vi "example async loop.vi"() -> ()   [LabVIEW 2016]
panel:
  out "data1 2":u32
  out "data1":u32
  out "packetType":T1(ring)
  out "System Index":u32
  in  "Channel":u32
  in  "Position Difference [nm]":i32=8000
  out "Error":errorcluster
  out "State":enum16{"POLL", "IDLE", "START", "RUN", "STOP"}(ring)
  in  "abort":bool
  out "Exit":bool
  out "connected":bool
  in  "connect":bool
  in  "findSystems":bool caption="Find Systems"
  in  "System locator":string(combo)
  in  "start":bool
  # "A linear positioner with integrated sensor \nshould be connected to channel 0."
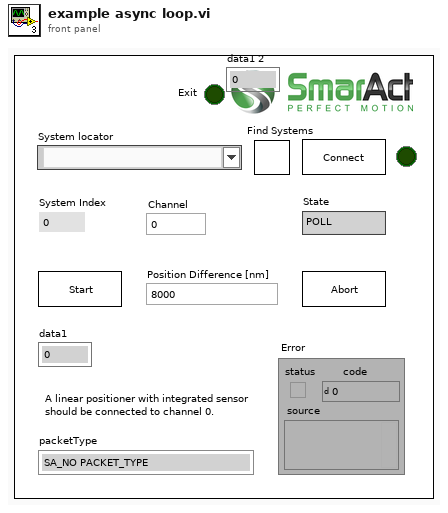
[diagram p1: front panel]
types:
  T1 = enum32{"SA_NO PACKET_TYPE", "SA_ERROR_ PACKET_TYPE", "SA_POSITION PACKET_TYPE", "SA_COMPLETED PACKET_TYPE", "SA_STATUS PACKET_TYPE", "SA_ANGLE_PACKET_TYPE", "SA_VOLTAGE_LEVEL_PACKET_TYPE", "SA_SENSOR_TYPE_PACKET_TYPE", "SA_SENSOR_ENABLED_PACKET_TYPE", "SA_END_EFFECTOR_TYPE_PACKET_TYPE", "SA_GRIPPER_OPENING_PACKET_TYPE", "SA_FORCE_PACKET_TYPE", "SA_MOVE_SPEED_PACKET_TYPE", "SA_PHYSICAL_POSITION_KNOWN_PACKET_TYPE", "SA_POSITION_LIMIT_PACKET_TYPE", "SA_ANGLE_LIMIT_PACKET_TYPE", "SA_SAFE_DIRECTION_PACKET_TYPE", "SA_SCALE_PACKET_TYPE", "SA_MOVE_ACCELERATION_PACKET_TYPE", "SA_CHANNEL_PROPERTY_PACKET_TYPE", "SA_CAPTURE_BUFFER_PACKET_TYPE", "SA_TRIGGERED_PACKET_TYPE"}
  T2 = enum32{"SA_NO_REPORT_ON_COMPLETE", "SA_REPORT_ON_COMPLETE"}
  T3 = enum32{"SA_SENSOR_DISABLED", "SA_SENSOR_ENABLED", "SA_SENSOR_POWERSAVE"}
  T4 = enum32{"SA_UNBUFFERED_OUTPUT", "SA_BUFFERED_OUTPUT"}
  T5 = typedef "mcsPacket.ctl" = cluster{"packetType":enum32{"SA_NO PACKET_TYPE", "SA_ERROR_ PACKET_TYPE", "SA_POSITION PACKET_TYPE", "SA_COMPLETED PACKET_TYPE", "SA_STATUS PACKET_TYPE", "SA_ANGLE_PACKET_TYPE", "SA_VOLTAGE_LEVEL_PACKET_TYPE", "SA_SENSOR_TYPE_PACKET_TYPE", "SA_SENSOR_ENABLED_PACKET_TYPE", "SA_END_EFFECTOR_TYPE_PACKET_TYPE", "SA_GRIPPER_OPENING_PACKET_TYPE", "SA_FORCE_PACKET_TYPE", "SA_MOVE_SPEED_PACKET_TYPE", "SA_PHYSICAL_POSITION_KNOWN_PACKET_TYPE", "SA_POSITION_LIMIT_PACKET_TYPE", "SA_ANGLE_LIMIT_PACKET_TYPE", "SA_SAFE_DIRECTION_PACKET_TYPE", "SA_SCALE_PACKET_TYPE", "SA_MOVE_ACCELERATION_PACKET_TYPE", "SA_CHANNEL_PROPERTY_PACKET_TYPE", "SA_CAPTURE_BUFFER_PACKET_TYPE", "SA_TRIGGERED_PACKET_TYPE"}, "channelIndex":u32, "data1":u32, "data2":i32, "data3":i32, "data4":u32}
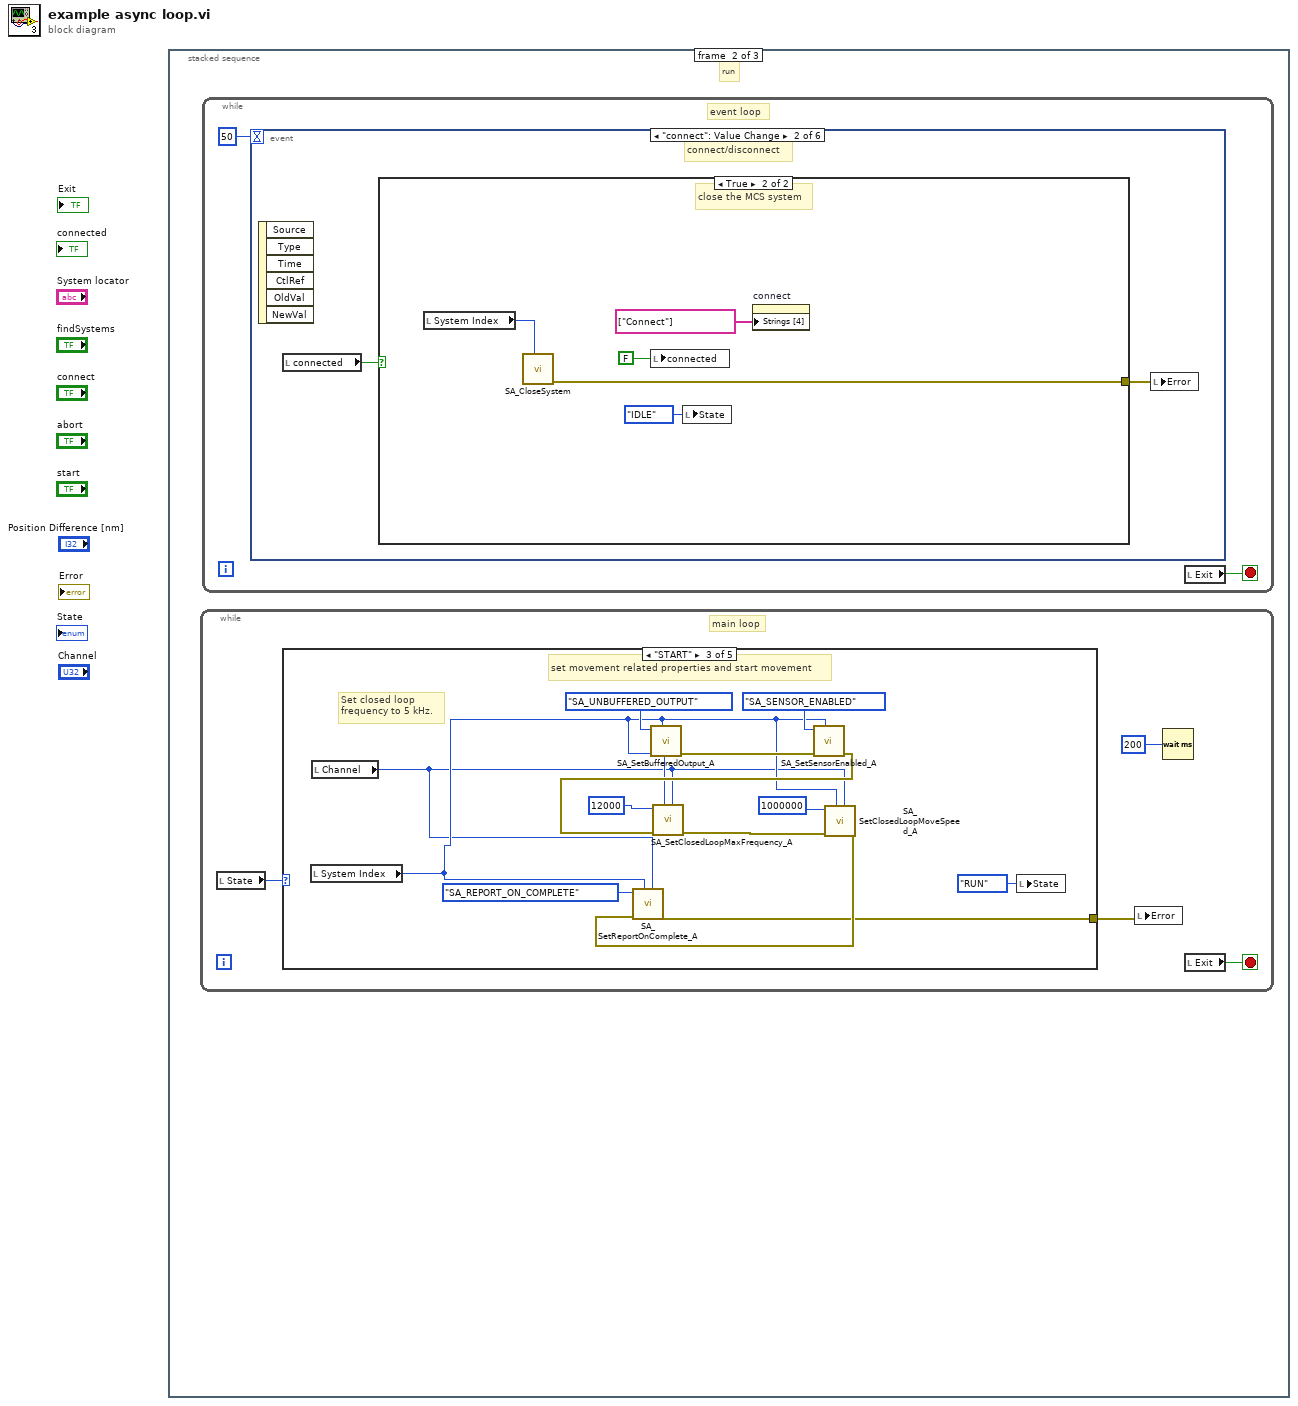
[diagram p0: block diagram]
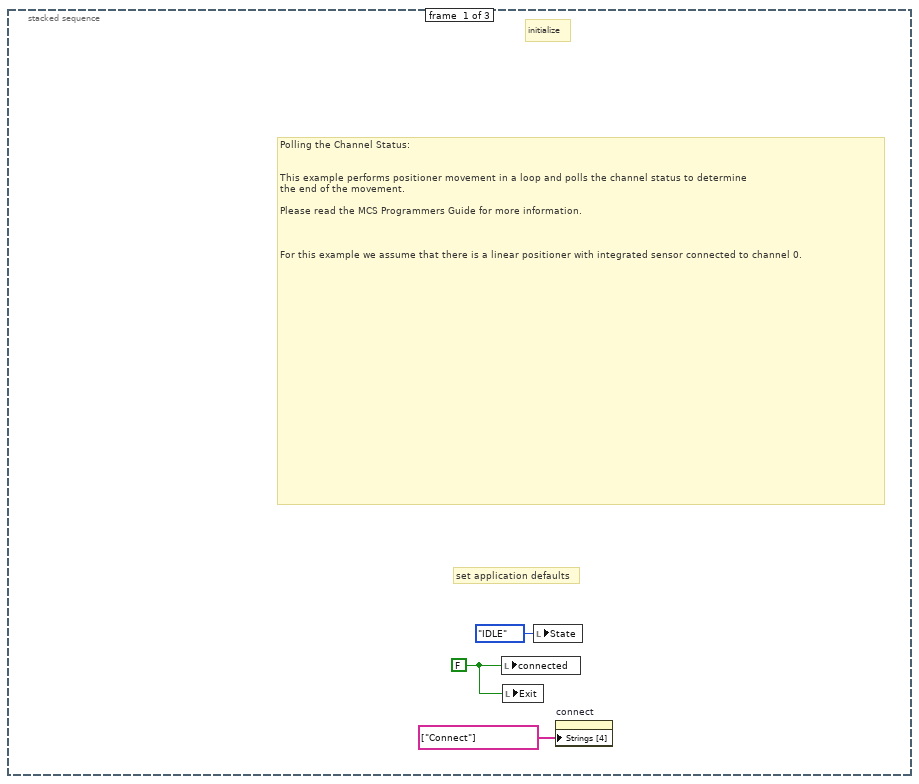
[diagram p2: hidden frame]
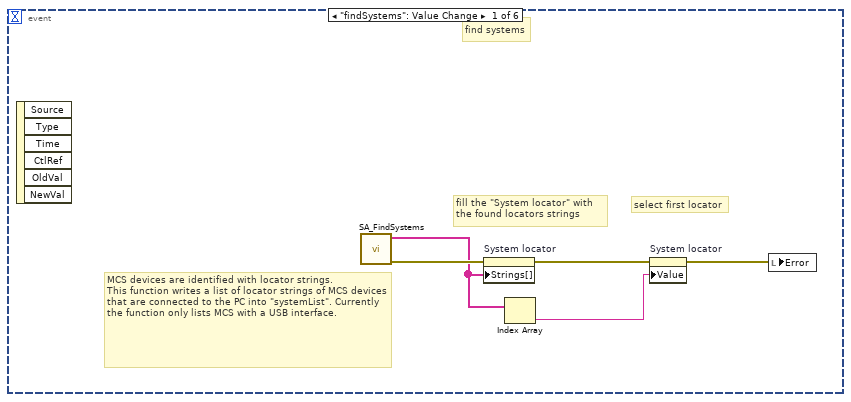
[diagram p3: hidden frame]
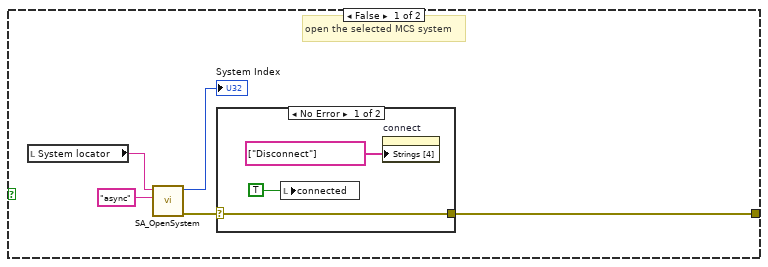
[diagram p4: hidden frame]
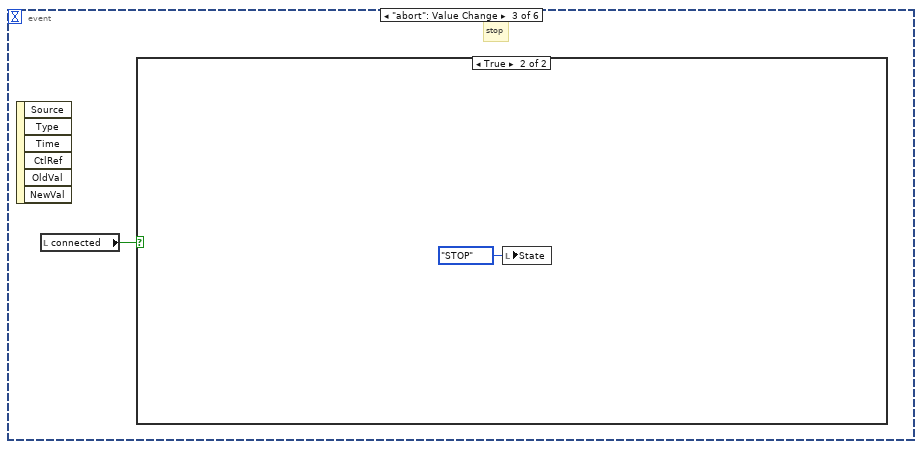
[diagram p6: hidden frame]
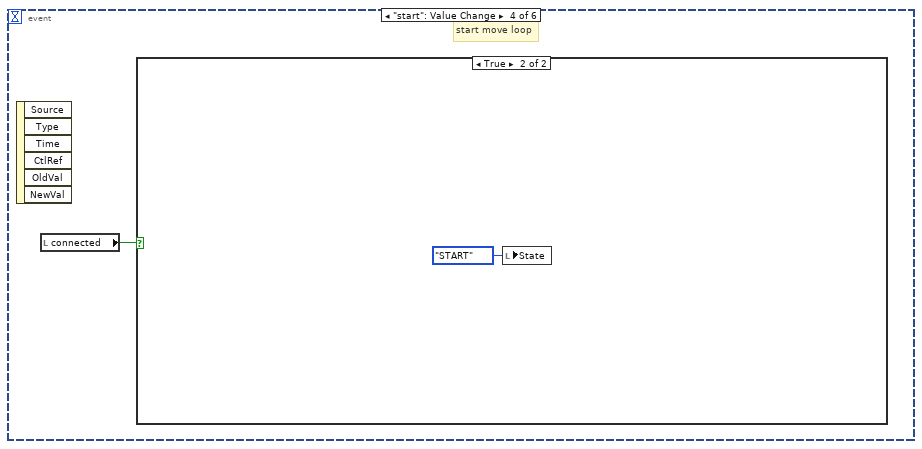
[diagram p8: hidden frame]
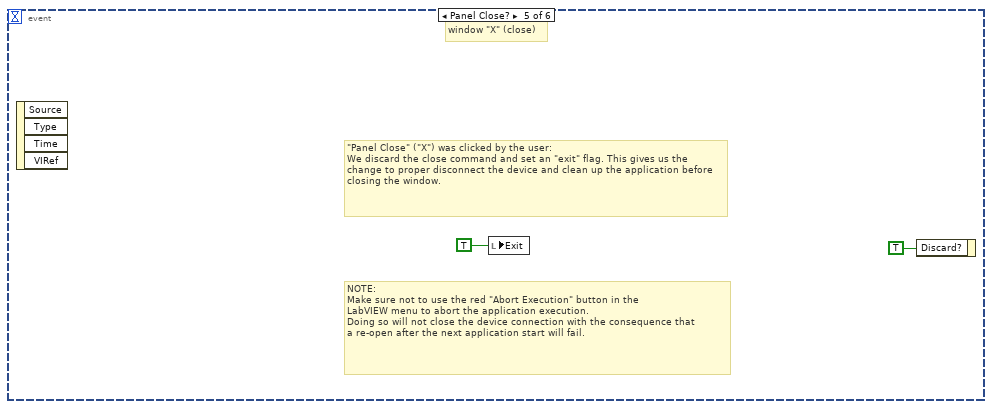
[diagram p10: hidden frame]
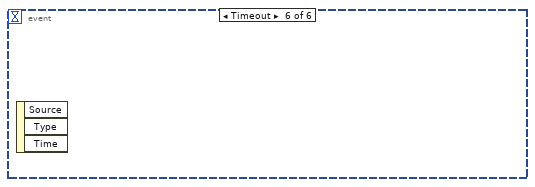
[diagram p11: hidden frame]
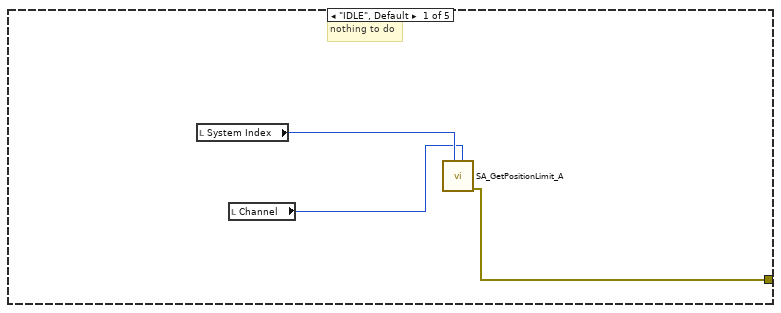
[diagram p12: hidden frame]
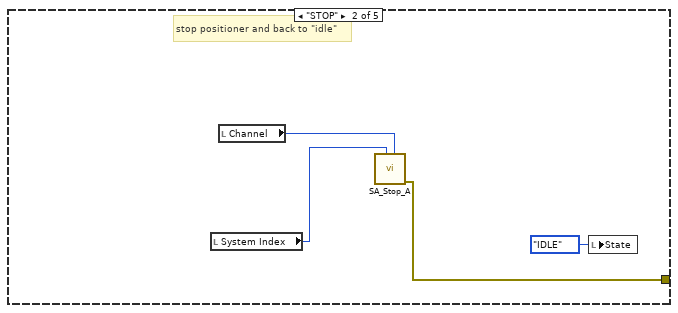
[diagram p13: hidden frame]
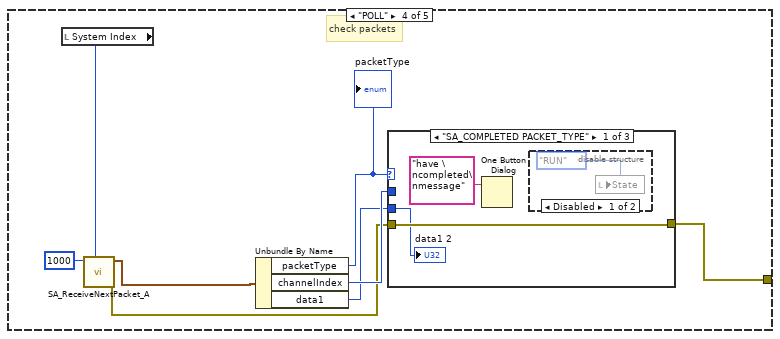
[diagram p14: hidden frame]
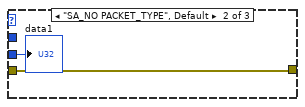
[diagram p16: hidden frame]
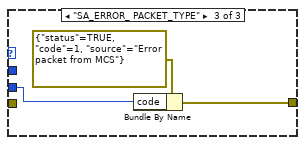
[diagram p17: hidden frame]
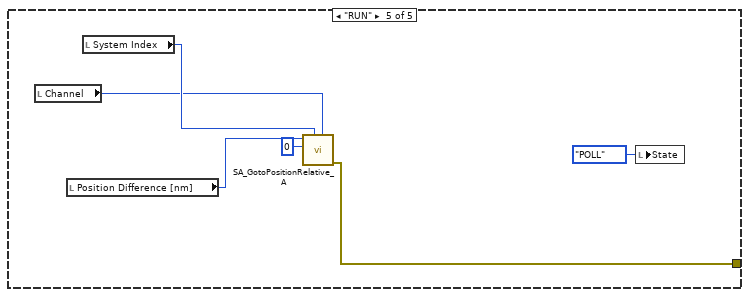
[diagram p18: hidden frame]
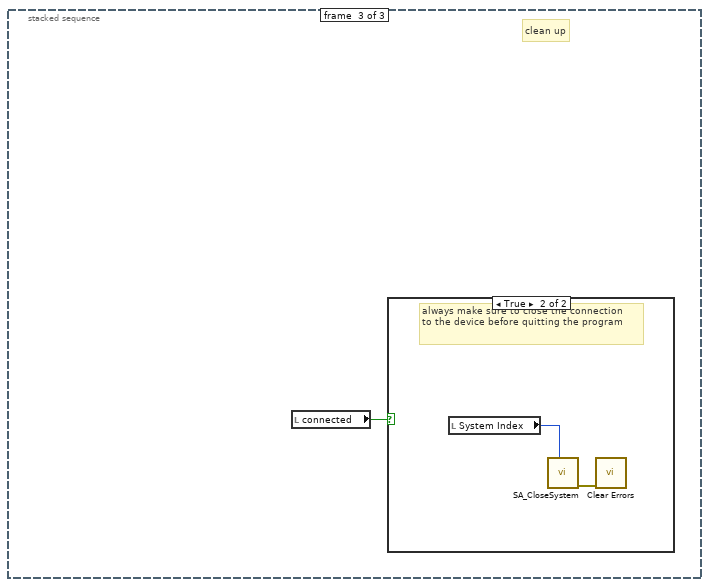
[diagram p19: hidden frame]
diagram:
  n1 = stacked-sequence {
    frame #0 {
      w3 = FALSE ("connected")
      # "Polling the Channel Status:\n\n\nThis example performs positioner movement in a loop and polls the channel status to determine\nthe end of the movement.\n\nPlease read the MCS Programmers Guide for more information.\n\n\n\nFor this example we assume that there is a linear positioner with integrated sensor connected to channel 0."
      # "set application defaults"
      # "initialize"
      n2 = local write "connected"(w3) -> ()
      n3 = local write "Exit"(w3) -> ()
      n4 = local write "State"(enum16{"POLL", "IDLE", "START", "RUN", "STOP"}."IDLE" ("State")) -> ()
      n5 = property on="connect" class="Bool"("Strings [4]"=string[] ["Connect"]) -> ()  [unwired: 2 in, 2 out]
    }
    frame #1 {
      # "run"
      n6 = while {
        stop <- w36 stop-if-true
        # "main loop"
        n7 = local read "State"() -> (w34:enum16{"POLL", "IDLE", "START", "RUN", "STOP"})
        n8 = case shown="\"START\"" w34 {
          tunnel: [w37 w42 w44 w58 w75] -> w33
          frame "IDLE", Default {
            # "nothing to do"
            n9 = local read "System Index"() -> (w39:u32)
            n10 = local read "Channel"() -> (w38:u32)
            n11 = call <vilib>:"SA_GetPositionLimit_A.vi"("channelIndex"=w38, "systemIndex"=w39) -> ("error out"=w37:errorcluster)  [unwired: 9 in]
          }
          frame "STOP" {
            # "stop positioner and back to \"idle\""
            n12 = local read "System Index"() -> (w41:u32)
            n13 = local read "Channel"() -> (w40:u32)
            n14 = call <vilib>:"SA_Stop_A.vi"("channelIndex"=w40, "systemIndex"=w41) -> ("error out"=w42:errorcluster)  [unwired: 9 in]
            n15 = local write "State"(enum16{"POLL", "IDLE", "START", "RUN", "STOP"}."IDLE" ("State")) -> ()
          }
          frame "START" {
            # "Set closed loop frequency to 5 kHz."
            # "set movement related properties and start movement"
            n16 = local read "System Index"() -> (w47:u32)
            n17 = local read "Channel"() -> (w46:u32)
            n18 = call <vilib>:"SA_SetBufferedOutput_A.vi"("systemIndex"=w47, "mode"=T4."SA_UNBUFFERED_OUTPUT") -> ("error out"=w54:errorcluster)  [unwired: 9 in]
            n19 = call <vilib>:"SA_SetSensorEnabled_A.vi"("systemIndex"=w47, "error in (no error)"=w54, "enabled"=T3."SA_SENSOR_ENABLED") -> ("error out"=w50:errorcluster)  [unwired: 8 in]
            n20 = call <vilib>:"SA_SetClosedLoopMaxFrequency_A.vi"("channelIndex"=w46, "systemIndex"=w47, "error in (no error)"=w50, "frequency"=u32 12000) -> ("error out"=w52:errorcluster)  [unwired: 7 in]
            n21 = call <vilib>:"SA_SetClosedLoopMoveSpeed_A.vi"("channelIndex"=w46, "systemIndex"=w47, "error in (no error)"=w52, "speed"=u32 1000000) -> ("error out"=w45:errorcluster)  [unwired: 7 in]
            n22 = call <vilib>:"SA_SetReportOnComplete_A.vi"("channelIndex"=w46, "systemIndex"=w47, "error in (no error)"=w45, "report"=T2."SA_REPORT_ON_COMPLETE") -> ("error out"=w44:errorcluster)  [unwired: 7 in]
            n23 = local write "State"(enum16{"POLL", "IDLE", "START", "RUN", "STOP"}."RUN" ("State")) -> ()
          }
          frame "POLL" {
            # "check packets"
            n24 = local read "System Index"() -> (w63:u32)
            n25 = call <vilib>:"SA_ReceiveNextPacket_A.vi"("systemIndex"=w63, "timeout"=u32 1000) -> ("error out"=w57:errorcluster, "packet"=w62:T5)  [unwired: 8 in]
            n26 = Unbundle By Name(w62) -> ("packetType"=w61:T1, "channelIndex"=w60:u32, "data1"=w59:u32)
            "packetType" <- w61
            n27 = case shown="\"SA_COMPLETED PACKET_TYPE\"" w61 {
              tunnel: [w67 w70 w72] -> w58
              tunnel: w59 -> [w65 w69 w71]
              tunnel: w60 -> [_ _ _]
              tunnel: w57 -> [w67 w70 _]
              frame "SA_COMPLETED PACKET_TYPE" {
                n28 = One Button Dialog(message="have \ncompleted\nmessage") -> ()  [unwired: 1 in, 1 out]
                n29 = disable-structure shown="Disabled" {
                  frame Disabled {
                    n30 = local write "State"(enum16{"POLL", "IDLE", "START", "RUN", "STOP"}."RUN" ("State")) -> ()
                  }
                  frame Enabled {
                  }
                }
                "data1 2" <- w65
              }
              frame "SA_NO PACKET_TYPE", Default {
                "data1" <- w69
              }
              frame "SA_ERROR_ PACKET_TYPE" {
                n31 = Bundle By Name(cluster=errorcluster {"status"=TRUE, "code"=1, "source"="Error packet from MCS"} ("error out"), "code"=w71) -> (w72:errorcluster)
              }
            }
          }
          frame "RUN" {
            n32 = local read "Channel"() -> (w77:u32)
            n33 = local read "Position Difference [nm]"() -> (w76:i32)
            n34 = local read "System Index"() -> (w78:u32)
            n35 = call <vilib>:"SA_GotoPositionRelative_A.vi"("channelIndex"=w77, "systemIndex"=w78, "holdTime"=u32 0, "diff"=w76) -> ("error out"=w75:errorcluster)  [unwired: 7 in]
            n36 = local write "State"(enum16{"POLL", "IDLE", "START", "RUN", "STOP"}."POLL" ("State")) -> ()
          }
        }
        n37 = local write "Error"(w33) -> ()
        n38 = Wait (ms)(milliseconds to wait=u32 200) -> ()  [unwired: 1 out]
        n39 = local read "Exit"() -> (w36:bool)
      }
      n40 = while {
        stop <- w4 stop-if-true
        # "event loop"
        n41 = event shown="[1] \"connect\": Value Change" {
          selector: _ -> [_ _ _ _ _ _]
          dyn-events: _ -> [_ _ _ _ _ _]
          timeout: 50 -> [_ _ _ _ _ _]
          event "findSystems": Value Change {
            # "select first locator"
            # "fill the \"System locator\" with\nthe found locators strings"
            # "MCS devices are identified with locator strings.\nThis function writes a list of locator strings of MCS devices that are connected to the PC into \"systemList\". Currently the function only lists MCS with a USB interface."
            # "find systems"
            n42 = event-data() -> ()  [unwired: 1 in, 6 out]
            n43 = call <vilib>:"SA_FindSystems.vi"() -> ("error out"=w10:errorcluster, "systemList"=w9:string[])  [unwired: 10 in]
            n44 = property on="System locator" class="CmbBox"(error in=w10, "Strings[]"=w9) -> (error out=w8:errorcluster)  [unwired: 1 in, 1 out]
            n45 = Index Array(array=w9) -> (element=w7:string)  [unwired: 1 in]
            n46 = property on="System locator" class="CmbBox"(error in=w8, "Value"=w7) -> (error out=w6:errorcluster)  [unwired: 1 in, 1 out]
            n47 = local write "Error"(w6) -> ()
          }
          event "connect": Value Change {
            # "connect/disconnect"
            n48 = event-data() -> ()  [unwired: 1 in, 6 out]
            n49 = local read "connected"() -> (w12:bool)
            n50 = case shown="True" w12 {
              tunnel: [w15 w23] -> w11
              frame False {
                # "open the selected MCS system"
                n51 = local read "System locator"() -> (w16:string)
                n52 = call <vilib>:"SA_OpenSystem.vi"("options"="async", "systemLocator"=w16) -> ("error out"=w17:errorcluster, "systemIndexOut"=→"System Index":u32)  [unwired: 8 in]
                n53 = case shown="No Error" w17 {
                  selector: w17 -> [w18 w21]
                  tunnel: [w18 w21] -> w15
                  frame No Error {
                    n54 = local write "connected"(TRUE ("connected")) -> ()
                    n55 = property on="connect" class="Bool"("Strings [4]"=string[] ["Disconnect"]) -> ()  [unwired: 2 in, 2 out]
                  }
                  frame Error {
                  }
                }
              }
              frame True {
                # "close the MCS system"
                n56 = local read "System Index"() -> (w26:u32)
                n57 = call <vilib>:"SA_CloseSystem.vi"("systemIndex"=w26) -> ("error out"=w23:errorcluster)  [unwired: 10 in]
                n58 = local write "connected"(FALSE ("connected")) -> ()
                n59 = local write "State"(enum16{"POLL", "IDLE", "START", "RUN", "STOP"}."IDLE" ("State")) -> ()
                n60 = property on="connect" class="Bool"("Strings [4]"=string[] ["Connect"]) -> ()  [unwired: 2 in, 2 out]
              }
            }
            n61 = local write "Error"(w11) -> ()
          }
          event "abort": Value Change {
            # "stop"
            n62 = event-data() -> ()  [unwired: 1 in, 6 out]
            n63 = local read "connected"() -> (w27:bool)
            n64 = case shown="True" w27 {
              frame False {
              }
              frame True {
                n65 = local write "State"(enum16{"POLL", "IDLE", "START", "RUN", "STOP"}."STOP" ("State")) -> ()
              }
            }
          }
          event "start": Value Change {
            # "start move loop"
            n66 = event-data() -> ()  [unwired: 1 in, 6 out]
            n67 = local read "connected"() -> (w29:bool)
            n68 = case shown="True" w29 {
              frame False {
              }
              frame True {
                n69 = local write "State"(enum16{"POLL", "IDLE", "START", "RUN", "STOP"}."START" ("State")) -> ()
              }
            }
          }
          event Panel Close? {
            # "NOTE:\nMake sure not to use the red \"Abort Execution\" button in the\nLabVIEW menu to abort the application execution.\nDoing so will not close the device connection with the consequence that\na re-open after the next application start will fail."
            # "\"Panel Close\" (\"X\") was clicked by the user:\nWe discard the close command and set an \"exit\" flag. This gives us the change to proper disconnect the device and clean up the application before closing the window."
            # "window \"X\" (close)"
            n70 = event-data() -> ()  [unwired: 1 in, 4 out]
            n71 = local write "Exit"(TRUE ("exit")) -> ()
            n72 = event-data("Discard?"=TRUE) -> ()  [unwired: 1 in, 1 out]
          }
          event Timeout {
            n73 = event-data() -> ()  [unwired: 1 in, 3 out]
          }
        }
        n74 = local read "Exit"() -> (w4:bool)
      }
    }
    frame #2 {
      # "clean up"
      n75 = local read "connected"() -> (w80:bool)
      n76 = case shown="True" w80 {
        frame False {
        }
        frame True {
          # "always make sure to close the connection\nto the device before quitting the program"
          n77 = local read "System Index"() -> (w82:u32)
          n78 = call <vilib>:"SA_CloseSystem.vi"("systemIndex"=w82) -> ("error out"=w81:errorcluster)  [unwired: 10 in]
          n79 = call <vilib>:"Clear Errors.vi"("error in (no error)"=w81) -> ()  [unwired: 5 in, 2 out]
        }
      }
    }
  }
